vi "ABF2_Read.vi"(4 "에러 입력":errorcluster, 7 "FilePath":path=path "C:/Users/KimYG/Experimental Data/Flocculus_Ex vivo/6. Plsticity/190119/190119_#07/190119__0026.abf") -> (0 "error out":errorcluster caption="에러 출력", 2 "DataProperties":T1, 3 "DataArray":sgl[][](array[numeric]))   [LabVIEW 2017]
uses:
  ABFFIO.lvclass
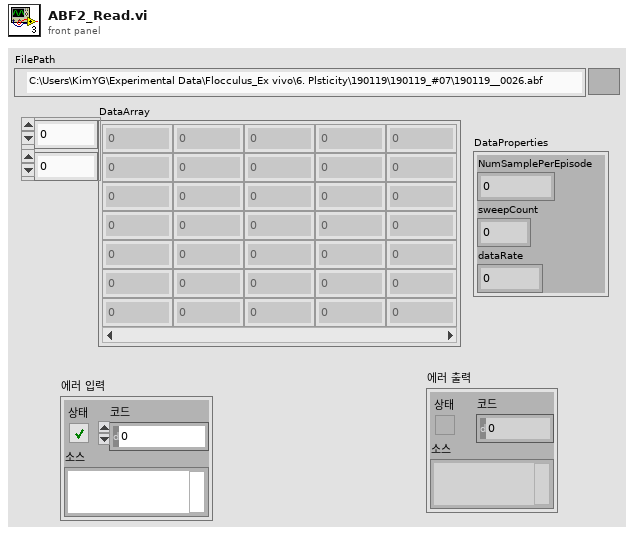
[diagram p1: front panel]
types:
  T1 = cluster{"NumSamplePerEpisode":u32, "sweepCount":u32, "dataRate":i32}
  T2 = enum16{"ProtocolSection", "ADCSection", "DACSection", "EpochSection", "ADCPerDACSection", "EpochPerDACSection", "StringsSection", "DataSection", "TagSection"}
  T3 = cluster{"blockNumber":u32, "byteCount":u32, "itemCount":u32}
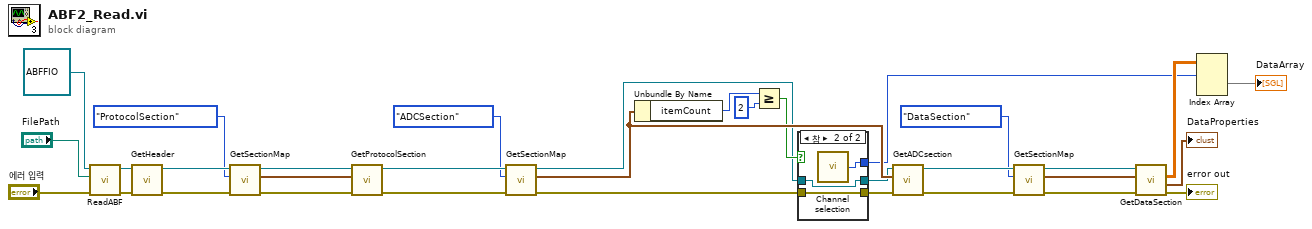
[diagram p0: block diagram]
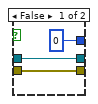
[diagram p2: hidden frame]
diagram:
  n1 = call "ReadABF.vi"("에러 입력"="에러 입력", "FilePath"="FilePath", "ABFFIO.lvclass IN"=refnum<class "ABFFIO.lvclass"> refnum) -> ("error out"=w30:errorcluster, "ABFFIO.lvclass OUT"=w31:refnum<class "ABFFIO.lvclass">)  [unwired: 3 in]
  n2 = call-dynamic "GetHeader.vi"("error in (no error)"=w30, "ABFFIO 입력"=w31) -> ("error out"=w28:errorcluster, "ABFFIO 출력"=w29:refnum<class "ABFFIO.lvclass">)  [unwired: 8 in]
  n3 = call-dynamic "GetSectionMap.vi"("error in (no error)"=w28, "Section"=T2."ProtocolSection", "ABFFIO 입력"=w29) -> ("error out"=w24:errorcluster, "SectionMap"=w26:T3, "ABFFIO 출력"=w25:refnum<class "ABFFIO.lvclass">)  [unwired: 6 in]
  n4 = call-dynamic "GetProtocolSection.vi"("error in (no error)"=w24, "SectionMap"=w26, "ABFFIO 입력"=w25) -> ("error out"=w22:errorcluster, "ABFFIO 출력"=w23:refnum<class "ABFFIO.lvclass">)  [unwired: 7 in]
  n5 = call-dynamic "GetSectionMap.vi"("error in (no error)"=w22, "Section"=T2."ADCSection", "ABFFIO 입력"=w23) -> ("error out"=w5:errorcluster, "SectionMap"=w11:T3, "ABFFIO 출력"=w7:refnum<class "ABFFIO.lvclass">)  [unwired: 6 in]
  n6 = Unbundle By Name(w11) -> ("itemCount"=w10:u32)
  n7 = Greater Or Equal?(x=w10, y=u32 2) -> (x >= y?=w8:bool)
  n8 = case shown="참" w8 {
    tunnel: w7 -> [w36 w39]
    tunnel: [w36 w39] -> w6
    tunnel: w5 -> [w35 w38]
    tunnel: [w35 w38] -> w4
    tunnel: [u16 0 ("channel") w37] -> w2
    frame False {
    }
    frame True {
      n9 = call "Channel selection.vi"() -> ("channel"=w37:u16)  [unwired: 1 in]
    }
  }
  n10 = call-dynamic "GetADCsection.vi"("error in (no error)"=w4, "SectionMap"=w11, "ABFFIO 입력"=w6) -> ("error out"=w19:errorcluster, "ABFFIO 출력"=w20:refnum<class "ABFFIO.lvclass">)  [unwired: 7 in]
  n11 = call-dynamic "GetSectionMap.vi"("error in (no error)"=w19, "Section"=T2."DataSection", "ABFFIO 입력"=w20) -> ("error out"=w15:errorcluster, "SectionMap"=w16:T3, "ABFFIO 출력"=w17:refnum<class "ABFFIO.lvclass">)  [unwired: 6 in]
  n12 = call-dynamic "GetDataSection.vi"("error in (no error)"=w15, "SectionMap"=w16, "ABFFIO 입력"=w17) -> ("error out"=→"error out":errorcluster, "DataProperties"=→"DataProperties":T1, "배열"=w3:sgl[][][])  [unwired: 5 in, 1 out]
  n13 = Index Array(array=w3, index (dim 0)=w2) -> (element=→"DataArray":sgl[][])  [unwired: 2 in]
